vi "Log.vi"(7 "Level":T1, 8 "error in":errorcluster, 9 "Error to Log":errorcluster, 10 "Message":string, 11 "Logger in":refnum<class "Logger.lvclass">) -> (0 "error out":errorcluster, 3 "Logger out":refnum<class "Logger.lvclass">)   [LabVIEW 2016, in "hse-logger.lvlib" / "Logger.lvclass"]
doc: "Creates a ``LogRecord`` with the specified level, message and error-cluster, und passes it to the registered ``Handlers``."
uses:
  Logger.lvclass
  LogLevel.ctl
  Logger.lvclass/Logger.ctl
  Handler/Handler.lvclass
  LogRecord/LogRecord.lvclass
  hse-logger.lvlib
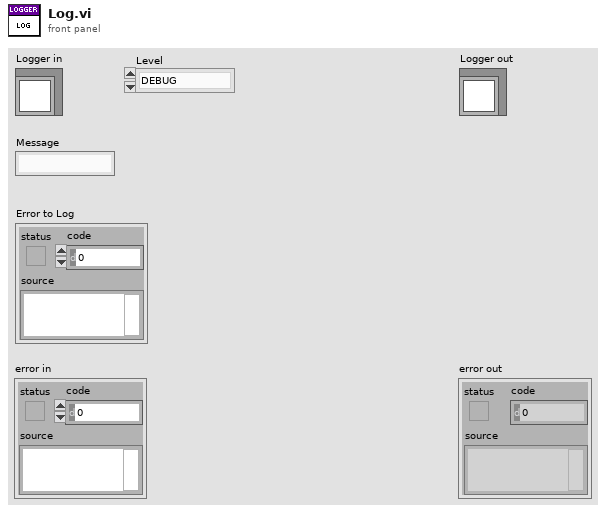
[diagram p1: front panel]
types:
  T1 = typedef "hse-logger.lvlib/LogLevel.ctl" = enum16{"DEBUG", "INFO", "WARNING", "ERROR", "CRITICAL"}
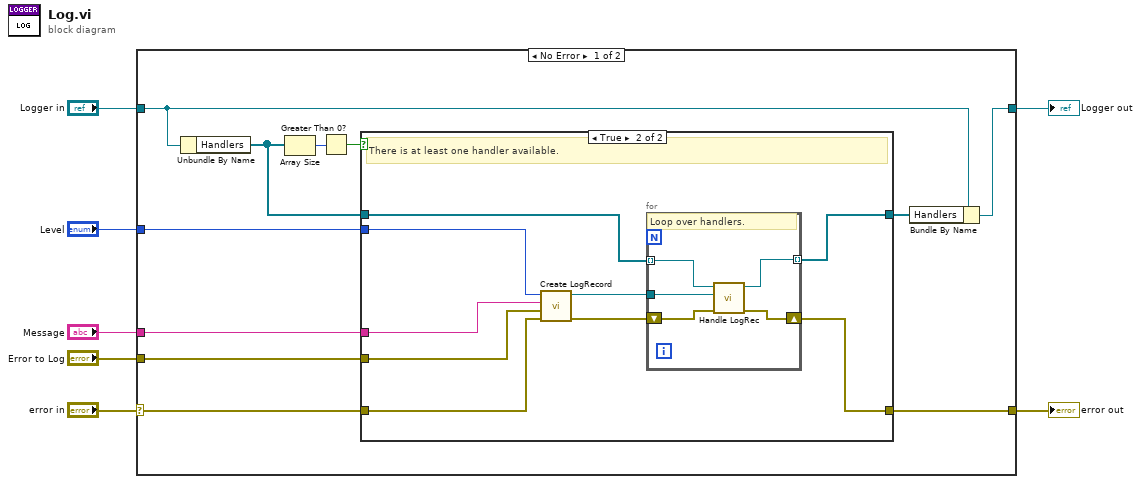
[diagram p0: block diagram]
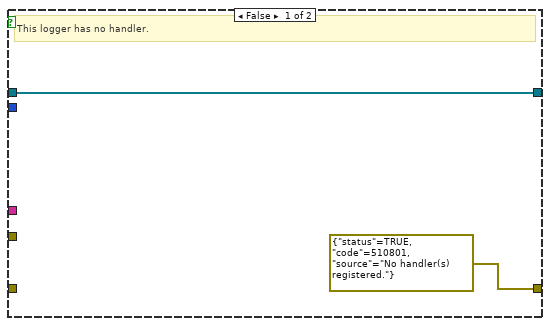
[diagram p2: hidden frame]
diagram:
  n1 = case shown="No Error" "error in" {
    selector: "error in" -> [w11 w36]
    tunnel: [w16 w36] -> w6
    tunnel: [w8 w35] -> w4
    tunnel: "Logger in" -> [w9 w35]
    tunnel: "Level" -> [w14 _]
    tunnel: "Message" -> [w13 _]
    tunnel: "Error to Log" -> [w12 _]
    frame No Error {
      n2 = Unbundle By Name(w9) -> ("Handlers"=w15:refnum<class "Handler.lvclass">[])
      n3 = Array Size(array=w15) -> (size(s)=w18:i32)
      n4 = Greater Than 0?(x=w18) -> (x > 0?=w17:bool)
      n5 = case shown="True" w17 {
        tunnel: [errorcluster {"status"=TRUE, "code"=510801, "source"="No handler(s) registered."} ("error IO") w29] -> w16
        tunnel: w15 -> [w20 w28]
        tunnel: w14 -> [_ w22]
        tunnel: w13 -> [_ w25]
        tunnel: w12 -> [_ w24]
        tunnel: w11 -> [_ w23]
        tunnel: [w20 w21] -> w10
        frame False {
          # "This logger has no handler."
        }
        frame True {
          # "There is at least one handler available."
          n6 = call "Create LogRecord.vi"("error in"=w23, "Error to Log"=w24, "Message"=w25, "Level"=w22) -> ("error out"=w26:errorcluster, "LogRecord out"=w27:refnum<class "LogRecord.lvclass">)  [unwired: 6 in]
          n7 = for {
            tunnel: w28 -> [w34] mode=indexing
            tunnel: w27 -> [w33]
            tunnel: [w30] -> w21 mode=indexing
            shift-right: [w31] -> w29
            shift-left: w26 -> [w32]
            # "Loop over handlers."
            n8 = call-dynamic "Handle LogRec.vi"("error in"=w32, "LogRecord"=w33, "Handler in"=w34) -> ("error out"=w31:errorcluster, "Handler out"=w30:refnum<class "Handler.lvclass">)  [unwired: 7 in]
          }
        }
      }
      n9 = Bundle By Name(cluster=w9, "Handlers"=w10) -> (w8:refnum<class "Logger.lvclass">)
    }
    frame Error {
    }
  }
  "error out" <- w6
  "Logger out" <- w4
